vi "ex14-12.vi"() -> ()   [LabVIEW 2014]
panel:
  in  "Y":dbl
  in  "X":dbl
  out "X移動Y位元":dbl format="%.3g"
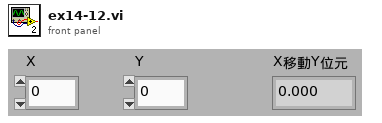
[diagram p1: front panel]
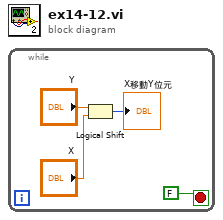
[diagram p0: block diagram]
diagram:
  n1 = while {
    stop <- FALSE stop-if-true
    n2 = Logical Shift(y="Y", x="X") -> (x << y=→"X移動Y位元":u32)
  }
